vi "New Project.vi"(9 "DBSet":T1={"Server"="172.20.23.107", "DB"="HTPSDB", "PSW"="data'songyy", "User"="sa"}, 10 "UserID":string="L043460", 11 "厂区":string="清溪") -> ()   [LabVIEW 2011] (continued)
                                n506 = local read "Luxshare_P/N:"() -> (w621:string)
                                n507 = local read "Luxshare_P/N:"() -> (w624:string)
                                n508 = local read "Luxshare_P/N:"() -> (w627:string)
                                n509 = local read "厂区"() -> ()  [unwired: 1 out]
                                n510 = local read "厂区"() -> (w583:string)
                                n511 = call "query.net.vi"() -> ()  [unwired: 10 in, 2 out]
                                n512 = call "_wmg_PNtoPNwhereConnect.vi"("Input"=w621) -> ("Output"=w595:string)
                                n513 = call "_wmg_PNtoPNwhereConnect.vi"("Input"=w627) -> ("Output"=w600:string)
                                n514 = call "_wmg_PNtoPNwhereConnect.vi"("Input"=w624) -> ("Output"=w598:string)
                                n515 = property on="System_Mode" class="Ring (严格)"() -> ("RingText.Text"=w594:string)  [unwired: 2 in, 2 out]
                                n516 = call "_wmg_HardModetoHardModewhereConnect.vi"("Input"=w594, "Factory"=w583) -> ("Output"=w585:string)
                                n517 = Concatenate Strings(w600, w585) -> (w599:string)
                                n518 = call "sql-readinfo_vproject.vi"("DBSet"=w582, "操作模式"=T7."查询数据", "查询项目"="Prjinf", "限定条件"=w599) -> ("ResultString"=w614:string)  [unwired: 13 in, 10 out]
                                n519 = local write "Project Information"(w614) -> ()
                                n520 = Concatenate Strings(w595, w585) -> (w593:string)
                                n521 = call "sql-readinfo_vproject.vi"("DBSet"=w582, "操作模式"=T7."查询数据", "查询项目"="SwitchMatrix", "限定条件"=w593) -> ("ResultString"=w616:string)  [unwired: 13 in, 10 out]
                                n522 = Concatenate Strings(w598, w585) -> (w597:string)
                                n523 = call "sql-readinfo_vproject.vi"("DBSet"=w582, "操作模式"=T7."查询数据", "查询项目"="Spec", "限定条件"=w597) -> ("ResultString"=→"Spec_midVar":string)  [unwired: 13 in, 10 out]
                                n524 = local write "Switch Matrix"(w616) -> ()
                                n525 = local read "Luxshare_P/N:"() -> (w606:string)
                                n526 = local read "Luxshare_P/N:"() -> (w609:string)
                                n527 = local read "Luxshare_P/N:"() -> (w612:string)
                                n528 = local read "Luxshare_P/N:"() -> (w618:string)
                                n529 = call "_wmg_PNtoPNwhereConnect.vi"("Input"=w606) -> ("Output"=w586:string)
                                n530 = Concatenate Strings(w586, w585) -> (w584:string)
                                n531 = call "_wmg_PNtoPNwhereConnect.vi"("Input"=w609) -> ("Output"=w588:string)
                                n532 = Concatenate Strings(w588, w585) -> (w587:string)
                                n533 = call "_wmg_PNtoPNwhereConnect.vi"("Input"=w612) -> ("Output"=w590:string)
                                n534 = Concatenate Strings(w590, w585) -> (w589:string)
                                n535 = call "sql-readinfo_vproject.vi"("DBSet"=w582, "操作模式"=T7."查询数据", "查询项目"="Spec_Points", "限定条件"=w584) -> ("ResultString"=w602:string)  [unwired: 13 in, 10 out]
                                n536 = call "sql-readinfo_vproject.vi"("DBSet"=w582, "操作模式"=T7."查询数据", "查询项目"="Switch_File_Path", "限定条件"=w589) -> ("ResultString"=w604:string)  [unwired: 13 in, 10 out]
                                n537 = call "_wmg_PNtoPNwhereConnect.vi"("Input"=w618) -> ("Output"=w592:string)
                                n538 = Concatenate Strings(w592, w585) -> (w591:string)
                                n539 = call "sql-readinfo_vproject.vi"("DBSet"=w582, "操作模式"=T7."查询数据", "查询项目"="LabelC", "限定条件"=w591) -> ("ResultString"=w615:string)  [unwired: 13 in, 10 out]
                                n540 = call "sql-readinfo_vproject.vi"("DBSet"=w582, "操作模式"=T7."查询数据", "查询项目"="Spec_File_Path", "限定条件"=w587) -> ("ResultString"=w603:string)  [unwired: 13 in, 10 out]
                                n541 = Decimal String To Number(string=w602) -> (number=w601:i32)  [unwired: 2 in, 1 out]
                                n542 = local write "Spec Points"(w601) -> ()
                                n543 = local write "Spec File Path"(w603) -> ()
                                n544 = local write "Switch File Path"(w604) -> ()
                                n545 = local write "Label Content"(w615) -> ()
                              }
                              frame Enabled {
                              }
                            }
                          }
                          frame #3 {
                            n546 = local read "Luxshare_P/N:"() -> (w644:string)
                            n547 = property on="System_Mode" class="Ring (严格)"() -> ("RingText.Text"=w643:string)  [unwired: 2 in, 2 out]
                            n548 = local read "厂区"() -> (w642:string)
                            n549 = Search and Replace String(input string="select SwitchMatrix ,Prjinf,Spec,LabelC,Switch_File_Path,Spec_File_Path,Spec_Points from vproject where LuxsharePN='@PN@' and HardWare_Mode='@Mode@' and  Factory ='@Facotry@'", search string="@PN@" ("搜索字符串"), replace string=w644) -> (result string=w648:string)  [unwired: 5 in, 3 out]
                            n550 = Search and Replace String(input string=w648, search string="@Mode@" ("搜索字符串"), replace string=w643) -> (result string=w646:string)  [unwired: 5 in, 3 out]
                            n551 = Search and Replace String(input string=w646, search string="@Facotry@" ("搜索字符串"), replace string=w642) -> (result string=w641:string)  [unwired: 5 in, 3 out]
                            n552 = call "query.net.vi"("Sql"=w641, "DBSet"=w640) -> ("result"=w639:string[][])  [unwired: 8 in, 1 out]
                            n553 = Index Array(array=w639, index (row)=0 ("索引 (行)")) -> (element=w637:string[])  [unwired: 1 in]
                            n554 = Index Array(array=w637) -> (element #1=w636:string, element #2=w635:string, element #3=w634:string, element #4=w633:string, element #5=w632:string, element #6=w631:string, element #7=w630:string)  [unwired: 7 in]
                            n555 = Decimal String To Number(string=w630) -> (number=w629:i32)  [unwired: 2 in, 1 out]
                            n556 = local write "Switch Matrix"(w636) -> ()
                            n557 = local write "Project Information"(w635) -> ()
                            n558 = local write "Spec_midVar"(w634) -> ()
                            n559 = local write "Label Content"(w633) -> ()
                            n560 = local write "Switch File Path"(w632) -> ()
                            n561 = local write "Spec File Path"(w631) -> ()
                            n562 = local write "Spec Points"(w629) -> ()
                          }
                          frame #4 {
                            n563 = control-ref of="Cable AWG:"() -> (w651:refnum<vi>)
                            n564 = local read "Spec_midVar"() -> (w654:string)
                            n565 = Search and Replace String(replace all?=TRUE ("替换全部？(F)"), input string=w654, search string="#" ("搜索字符串"), replace string="\t") -> (result string=w658:string)  [unwired: 4 in, 3 out]
                            n566 = control-ref of="Customer"() -> (w652:refnum<vi>)
                            n567 = local read "Customer"() -> (w665:string)
                            n568 = local read "AWG"() -> (w664:string)
                            n569 = Spreadsheet String To Array(format string="%s" ("格式字符串"), spreadsheet string=w658, array type (2D Dbl)=string[][] []) -> (array=w653:string[][])  [unwired: 1 in]
                            n570 = call "_wmg_downlistValue.vi"("Customer"=w664, "CustomerRef"=w651) -> ()  [unwired: 1 in]
                            n571 = call "_wmg_downlistValue.vi"("Customer"=w665, "CustomerRef"=w652) -> ()  [unwired: 1 in]
                            n572 = Array To Spreadsheet String(delimiter (Tab)="#" ("分隔符(Tab)"), array=w653, 3:"%s" ("格式字符串")) -> (spreadsheet string=w663:string)
                            n573 = local write "Spec Associate"(w653) -> ()
                            n574 = local write "Spec String"(w663) -> ()
                          }
                        }
                      }
                    }
                  }
                  frame #1 {
                    # "列数\n0. S-para Pair Name\n1. NEXT Pair Name\n2. FEXT Pair Name\n3. Diff TestItems\n4. Single TestItems\n5. TDR TestItems\n6. Spec Associate\n7. VNA Cal File Path\n8. Report Config\n9. ILD Spec\n10. TDR Setting"
                    # "解析Prjinf"
                    n575 = local read "Project Information"() -> (w700:string)
                    n576 = Spreadsheet String To Array(delimiter (Tab)="#" ("分隔符(Tab)"), format string="%s" ("格式字符串"), spreadsheet string=w700, array type (2D Dbl)=string[][] []) -> (array=w697:string[][])
                    n577 = Index Array(array=w697, index (col) #1=0 ("索引"), index (col) #2=1 ("索引 (列)"), index (col) #3=2 ("索引 (列)"), index (col) #4=3 ("索引 (列)"), index (col) #5=4 ("索引 (列)"), index (col) #6=5 ("索引"), index (col) #7=6 ("索引 (列)"), index (col) #8=7 ("索引 (列)"), index (col) #9=8 ("索引 (列)"), index (col) #10=9 ("索引 (列)"), index (col) #11=10 ("索引"), index (col) #12=11 ("索引 (列)"), index (col) #13=12 ("索引 (列)"), index (col) #14=13 ("索引 (列)"), index (col) #15=14 ("索引 (列)")) -> (element #1=w696:string[], element #2=w695:string[], element #3=w694:string[], element #4=w693:string[], element #5=w692:string[], element #6=w691:string[], element #7=w690:string[], element #8=w689:string[], element #9=w688:string[], element #10=w687:string[], element #11=w686:string[], element #12=w673:string[], element #13=w670:string[], element #14=w668:string[], element #15=w666:string[])  [unwired: 15 in]
                    n578 = stacked-sequence {
                      tunnel: w696 -> [_ w714 _ _ _ _ _ _ _]
                      tunnel: w695 -> [_ w713 _ _ _ _ _ _ _]
                      tunnel: w694 -> [_ w712 _ _ _ _ _ _ _]
                      tunnel: w693 -> [_ w711 _ _ _ _ _ _ _]
                      tunnel: w692 -> [_ w710 _ _ _ _ _ _ _]
                      tunnel: w691 -> [_ w709 _ _ _ _ _ _ _]
                      tunnel: w690 -> [_ _ w760 _ _ _ _ _ _]
                      tunnel: w689 -> [_ _ w759 _ _ _ _ _ _]
                      tunnel: w688 -> [_ _ _ w788 _ _ _ _ _]
                      tunnel: w687 -> [_ _ _ _ _ _ _ _ _]
                      tunnel: w686 -> [_ _ _ _ _ w808 _ _ _]
                      tunnel: w673 -> [_ _ _ _ _ _ w838 _ _]
                      tunnel: w670 -> [_ _ _ w780 _ _ _ _ _]
                      tunnel: w668 -> [_ _ _ _ _ _ _ w882 _]
                      tunnel: w666 -> [_ _ _ _ _ _ _ _ w889]
                      frame #0 {
                        n579 = local read "Single init"() -> (→"Single init 2":i32[])
                        n580 = local read "NEXT init"() -> (→"NEXT init 2":i32[])
                        n581 = local read "FEXT init"() -> (→"FEXT init 2":i32[])
                        n582 = local read "S-p init"() -> (→"S-p init 2":i32[])
                        n583 = local read "Diff init"() -> (→"Diff init 2":i32[])
                        n584 = local read "TDR init"() -> (→"TDR init 2":i32[])
                      }
                      frame #1 {
                        n585 = stacked-sequence {
                          tunnel: [_ w736 _ _] -> _
                          tunnel: w714 -> [_ w736 _ _]
                          tunnel: w713 -> [_ w729 _ _]
                          tunnel: w712 -> [_ _ w742 _]
                          tunnel: w711 -> [_ _ w737 _]
                          tunnel: w710 -> [_ _ _ w750]
                          tunnel: w709 -> [_ _ _ w747]
                          frame #0 {
                            n586 = local read "FEXT init"() -> (w722:string[])
                            n587 = local read "FEXT init"() -> (w721:i32[])
                            n588 = local read "NEXT init"() -> (w725:string[])
                            n589 = local read "NEXT init"() -> (w723:i32[])
                            n590 = local read "S-p init"() -> (w724:i32[])
                            n591 = local read "S-p init"() -> (w726:string[])
                            n592 = property on="S-para Pair Name" class="LstBox (严格)"("Item Names"=w726, "Item Symbols"=w724) -> ()  [unwired: 2 in, 2 out]
                            n593 = property on="NEXT Pair Name" class="LstBox (严格)"("Item Names"=w725, "Item Symbols"=w723) -> ()  [unwired: 2 in, 2 out]
                            n594 = property on="FEXT Pair Name" class="LstBox (严格)"("Item Names"=w722, "Item Symbols"=w721) -> ()  [unwired: 2 in, 2 out]
                            n595 = local read "Single init"() -> (w718:string[])
                            n596 = local read "Single init"() -> (w717:i32[])
                            n597 = local read "TDR init"() -> (w716:string[])
                            n598 = local read "TDR init"() -> (w715:i32[])
                            n599 = local read "Diff init"() -> (w720:string[])
                            n600 = local read "Diff init"() -> (w719:i32[])
                            n601 = property on="Diff Test Items" class="LstBox (严格)"("Item Names"=w720, "Item Symbols"=w719) -> ()  [unwired: 2 in, 2 out]
                            n602 = property on="Single Test Items" class="LstBox (严格)"("Item Names"=w718, "Item Symbols"=w717) -> ()  [unwired: 2 in, 2 out]
                            n603 = property on="TDR Test Items" class="LstBox (严格)"("Item Names"=w716, "Item Symbols"=w715) -> ()  [unwired: 2 in, 2 out]
                          }
                          frame #1 {
                            n604 = local read "S-p init"() -> (w734:i32[])
                            n605 = local read "NEXT init"() -> (w727:string[])
                            n606 = local read "NEXT init"() -> (w730:i32[])
                            n607 = local read "S-p init"() -> (w728:string[])
                            n608 = call "_wmg_readItems.vi"("input_p"=w734, "input"=w728, "input_sp"=w736) -> ("output_p"=w733:i32[], "output_sp"=w735:string[])
                            n609 = call "_wmg_readItems2.vi"("input_p"=w730, "input"=w727, "input_sp"=w729) -> ("output_p"=w731:i32[], "output_sp"=w732:string[])
                            n610 = property on="S-para Pair Name" class="LstBox (严格)"("Item Names"=w735, "Item Symbols"=w733) -> ()  [unwired: 2 in, 2 out]
                            n611 = property on="NEXT Pair Name" class="LstBox (严格)"("Item Names"=w732, "Item Symbols"=w731) -> ()  [unwired: 2 in, 2 out]
                          }
                          frame #2 {
                            n612 = local read "FEXT init"() -> (w745:string[])
                            n613 = local read "FEXT init"() -> (w746:i32[])
                            n614 = local read "Diff init"() -> (w741:string[])
                            n615 = local read "Diff init"() -> (w740:i32[])
                            n616 = call "_wmg_readItems2.vi"("input_p"=w740, "input"=w741, "input_sp"=w737) -> ("output_p"=w739:i32[], "output_sp"=w738:string[])
                            n617 = call "_wmg_readItems.vi"("input_p"=w746, "input"=w745, "input_sp"=w742) -> ("output_p"=w743:i32[], "output_sp"=w744:string[])
                            n618 = property on="FEXT Pair Name" class="LstBox (严格)"("Item Names"=w744, "Item Symbols"=w743) -> ()  [unwired: 2 in, 2 out]
                            n619 = property on="Diff Test Items" class="LstBox (严格)"("Item Names"=w738, "Item Symbols"=w739) -> ()  [unwired: 2 in, 2 out]
                          }
                          frame #3 {
                            n620 = local read "TDR init"() -> (w749:string[])
                            n621 = local read "TDR init"() -> (w748:i32[])
                            n622 = local read "Single init"() -> (w751:string[])
                            n623 = local read "Single init"() -> (w752:i32[])
                            n624 = call "_wmg_readItems.vi"("input_p"=w752, "input"=w751, "input_sp"=w750) -> ("output_p"=w754:i32[], "output_sp"=w753:string[])
                            n625 = call "_wmg_readItems2.vi"("input_p"=w748, "input"=w749, "input_sp"=w747) -> ("output_p"=w756:i32[], "output_sp"=w755:string[])
                            n626 = property on="TDR Test Items" class="LstBox (严格)"("Item Names"=w755, "Item Symbols"=w756) -> ()  [unwired: 2 in, 2 out]
                            n627 = property on="Single Test Items" class="LstBox (严格)"("Item Names"=w753, "Item Symbols"=w754) -> ()  [unwired: 2 in, 2 out]
                          }
                        }
                      }
                      frame #2 {
                        n628 = disable-structure shown="禁用" {
                          disable-tunnel: w760 -> [w761 _]
                          frame Disabled {
                            n629 = property on="Diff Test Items" class="LstBox (严格)"() -> ("Item Symbols"=w765:i32[], "Item Names"=w763:string[])  [unwired: 2 in, 2 out]
                            n630 = for {
                              tunnel: w765 -> [w771] mode=indexing
                              shift-right: [w766] -> w762
                              shift-left: string[] [] -> [w767]
                              tunnel: w763 -> [w768] mode=indexing
                              n631 = Not Equal?(x=w771, y=37) -> (x != y?=w769:bool)
                              n632 = case shown="假" w769 {
                                tunnel: w768 -> [_ w775]
                                tunnel: w767 -> [w772 w774]
                                tunnel: [w772 w773] -> w766
                                frame False {
                                }
                                frame True {
                                n633 = Insert Into Array(array=w774, new element=w775) -> (w773:string[])  [unwired: 1 in]
                                }
                              }
                            }
                            n634 = Build Array(w762, w761) -> ()  [unwired: 1 out]
                          }
                          frame Enabled {
                          }
                        }
                        n635 = Index Array(array=w759, index=0 ("索引")) -> (element=w758:string)
                        n636 = local write "VNA Cal File Path:"(w758) -> ()
                      }
                      frame #3 {
                        n637 = Index Array(array=w780, index=0 ("索引")) -> (element=w778:string)
                        n638 = Index Array(array=w788, index #1=0 ("索引"), index #3=2 ("索引")) -> (element #1=w785:string, element #2=w784:string, element #3=w782:string)  [unwired: 1 in]
                        n639 = Equal?(x=w778, y="TRUE") -> (x = y?=w776:bool)
                        n640 = String To Path(string=w785) -> (path=w786:path)
                        n641 = call "_wmg_ReportConfigDivided@.vi"("Input"=w784) -> ("Output"=w783:string[][])
                        n642 = call "_wmg_ReportConfigDivided@.vi"("Input"=w782) -> ("Output"=w781:string[][])
                        n643 = local write "Postion for Raw data"(w783) -> ()
                        n644 = local write "Report Templete Path:"(w786) -> ()
                        n645 = local write "Postion for \"PN&Tester&Date\" etc Fields"(w781) -> ()
                        n646 = local write "Cancel Dem2X?"(w776) -> ()
                      }
                      frame #4 {
                      }
                      frame #5 {
                        # "TDR Setting\n0. Start TimeNs\n1. Stop TimeNs\n2. Data Points\n3. Filter Risetime(ps)\n4. Compensation(ohm)\n5. Impedance Filter\n6. Impedance Spec:\n7. Delay Spec:\n8. skew Spec:\n9. IL 2X Data:"
                        n647 = Index Array(array=w808, index #1=0 ("索引"), index #2=1 ("索引"), index #3=2 ("索引"), index #4=3 ("索引"), index #5=4 ("索引"), index #6=5 ("索引"), index #7=6 ("索引"), index #8=9 ("索引"), index #9=8 ("索引")) -> (element #1=w800:string, element #2=w799:string, element #3=w798:string, element #4=w797:string, element #5=w796:string, element #6=w795:string, element #7=w794:string, element #8=w792:string, element #9=w790:string)
                        n648 = stacked-sequence {
                          tunnel: w800 -> [w835]
                          tunnel: w799 -> [w832]
                          tunnel: w798 -> [w830]
                          tunnel: w797 -> [w829]
                          tunnel: w796 -> [w826]
                          tunnel: w795 -> [w825]
                          tunnel: w794 -> [w822]
                          tunnel: w792 -> [w817]
                          tunnel: w790 -> [w811]
                          frame #0 {
                            n649 = call "_wmg_ImpSpecDivided@.vi"("Input"=w822) -> ("Output"=w821:string[][])
                            n650 = Spreadsheet String To Array(format string="%s" ("格式字符串"), spreadsheet string=w817, array type (2D Dbl)=dbl[] []) -> (array=w812:dbl[])  [unwired: 1 in]
                            n651 = Fract/Exp String To Number(string=w811) -> (number=w810:dbl)  [unwired: 3 in, 1 out]
                            n652 = local write "Skew max(ps)"(w810) -> ()
                            n653 = Insert Into Array(array=w821, index (col)=0 ("禁用的索引 (列)"), new element=string[] ["Mating Area", "Cable Area", "Cable End"]) -> (w819:string[][])  [unwired: 1 in]
                            n654 = local write "2X Thru  IL Data"(w812) -> ()
                            n655 = Decimal String To Number(string=w825) -> (number=w809:i32)  [unwired: 2 in, 1 out]
                            n656 = local write "Impedance Spec:"(w819) -> ()
                            n657 = Number To Boolean Array(number=w809) -> (Boolean array=w824:bool[])
                            n658 = Array To Spreadsheet String(array=w812, 3:"%s" ("格式字符串")) -> (spreadsheet string=w814:string)  [unwired: 1 in]
                            n659 = Fract/Exp String To Number(string=w826) -> (number=w827:dbl)  [unwired: 3 in, 1 out]
                            n660 = Index Array(array=w824) -> (element=w823:bool)  [unwired: 1 in]
                            n661 = Fract/Exp String To Number(string=w832) -> (number=w833:dbl)  [unwired: 3 in, 1 out]
                            n662 = Decimal String To Number(string=w830) -> (number=w831:i32)  [unwired: 2 in, 1 out]
                            n663 = Fract/Exp String To Number(string=w829) -> (number=w828:dbl)  [unwired: 3 in, 1 out]
                            n664 = local write "2X Thru String"(w814) -> ()
                            n665 = local write "Compensation(ohm)"(w827) -> ()
                            n666 = Fract/Exp String To Number(string=w835) -> (number=w834:dbl)  [unwired: 3 in, 1 out]
                            n667 = local write "Filter Risetime(ps)"(w828) -> ()
                            n668 = local write "Impedance Filter"(w823) -> ()
                            n669 = local write "Start TimeNs"(w834) -> ()
                            n670 = local write "StopTimeNs"(w833) -> ()
                            n671 = local write "Data Points"(w831) -> ()
                          }
                        }
                      }
                      frame #6 {
                        # "TDR Setting\n0. Start TimeNs\n1. Stop TimeNs\n2. Data Points\n3. Filter Risetime(ps)\n4. Compensation(ohm)\n5. Impedance Filter\n6. Impedance Spec:\n7. Delay Spec:\n8. skew Spec:\n9. IL 2X Data:"
                        n672 = Index Array(array=w838, index #1=0 ("索引"), index #2=1 ("索引"), index #3=2 ("索引"), index #4=3 ("索引"), index #5=4 ("索引"), index #6=5 ("索引"), index #7=6 ("索引"), index #8=9 ("索引"), index #9=8 ("索引")) -> (element #1=w847:string, element #2=w846:string, element #3=w845:string, element #4=w844:string, element #5=w843:string, element #6=w842:string, element #7=w841:string, element #8=w839:string, element #9=w836:string)
                        n673 = stacked-sequence {
                          tunnel: w847 -> [w878]
                          tunnel: w846 -> [w877]
                          tunnel: w845 -> [w876]
                          tunnel: w844 -> [w875]
                          tunnel: w843 -> [w874]
                          tunnel: w842 -> [w873]
                          tunnel: w841 -> [w871]
                          tunnel: w839 -> [w868]
                          tunnel: w836 -> [w858]
                          frame #0 {
                            (unwired) string[] ["Mating Area", "Cable Area"]
                            n674 = call "_wmg_ImpSpecDivided@.vi"("Input"=w871) -> ("Output"=w870:string[][])
                            n675 = Spreadsheet String To Array(format string="%s" ("格式字符串"), spreadsheet string=w868, array type (2D Dbl)=dbl[] []) -> ()  [unwired: 1 in, 1 out]
                            n676 = Fract/Exp String To Number(string=w858) -> (number=w857:dbl)  [unwired: 3 in, 1 out]
                            n677 = local write "Skew max(ps) 2"(w857) -> ()
                            n678 = Insert Into Array(array=w870, index (col)=0 ("禁用的索引 (列)"), new element=string[] ["Mating Area", "Cable Area", "Cable End"]) -> (w865:string[][])  [unwired: 1 in]
                            n679 = Decimal String To Number(string=w873) -> (number=w856:i32)  [unwired: 2 in, 1 out]
                            n680 = local write "Impedance Spec: 2"(w865) -> ()
                            n681 = Number To Boolean Array(number=w856) -> (Boolean array=w872:bool[])
                            n682 = Fract/Exp String To Number(string=w874) -> (number=w863:dbl)  [unwired: 3 in, 1 out]
                            n683 = Index Array(array=w872) -> (element=w864:bool)  [unwired: 1 in]
                            n684 = Fract/Exp String To Number(string=w877) -> (number=w860:dbl)  [unwired: 3 in, 1 out]
                            n685 = Decimal String To Number(string=w876) -> (number=w861:i32)  [unwired: 2 in, 1 out]
                            n686 = Fract/Exp String To Number(string=w875) -> (number=w862:dbl)  [unwired: 3 in, 1 out]
                            n687 = local write "Compensation(ohm) 2"(w863) -> ()
                            n688 = Fract/Exp String To Number(string=w878) -> (number=w859:dbl)  [unwired: 3 in, 1 out]
                            n689 = local write "Filter Risetime(ps) 2"(w862) -> ()
                            n690 = local write "Impedance Filter 2"(w864) -> ()
                            n691 = local write "Data Points 2"(w861) -> ()
                            n692 = local write "StopTimeNs 2"(w860) -> ()
                            n693 = local write "Start TimeNs 2"(w859) -> ()
                          }
                        }
                      }
                      frame #7 {
                        n694 = Index Array(array=w882, index=0 ("索引")) -> (element=w880:string)
                        n695 = Decimal String To Number(string=w880) -> (number=w879:i32)  [unwired: 2 in, 1 out]
                        n696 = local write "平滑点数"(w879) -> ()
                      }
                      frame #8 {
                        n697 = Index Array(array=w889, index=0 ("索引")) -> (element=w887:string)
                        n698 = call "_wmg_ImpSpecDivided@.vi"("Input"=w887) -> ("Output"=w886:string[][])
                        n699 = Insert Into Array(array=w886, index (col)=0 ("禁用的索引 (列)"), new element=string[] ["Mating Area", "Cable Area", "Cable End"]) -> (w883:string[][])  [unwired: 1 in]
                        n700 = local write "Common Impedance Spec"(w883) -> ()
                      }
                    }
                    n701 = disable-structure shown="禁用" {
                      frame Disabled {
                        n702 = local read "2X Thru  IL Data"() -> ()  [unwired: 1 in]
                        n703 = Array To Spreadsheet String(3:"%s" ("格式字符串")) -> (spreadsheet string=w701:string)  [unwired: 2 in]
                        n704 = local write "2X Thru String"(w701) -> ()
                      }
                      frame Enabled {
                      }
                    }
                  }
                  frame #2 {
                    w898 = T4 {"Row"=0, "Column"=0} ("编辑位置")
                    w899 = u32 4 ("列数")
                    n705 = property on="Single Test Items" class="LstBox (严格)"() -> ("Item Names"=w906:string[], "Item Symbols"=w905:i32[])  [unwired: 2 in, 2 out]
                    n706 = property on="TDR Test Items" class="LstBox (严格)"() -> ("Item Names"=w904:string[], "Item Symbols"=w903:i32[])  [unwired: 2 in, 2 out]
                    n707 = property on="Diff Test Items" class="LstBox (严格)"() -> ("Item Names"=w908:string[], "Item Symbols"=w907:i32[])  [unwired: 2 in, 2 out]
                    n708 = call "_wmg_SelectItems2.vi"("Item Syms"=w903, "Item name"=w904) -> ("Selected tem"=w902:string[])  [unwired: 7 in, 2 out]
                    n709 = call "_wmg_SelectItems2.vi"("Item Syms"=w907, "Item name"=w908) -> ("Selected tem"=w901:string[])  [unwired: 7 in, 2 out]
                    n710 = call "_wmg_SelectItems2.vi"("Item Syms"=w905, "Item name"=w906) -> ("Selected tem"=w900:string[])  [unwired: 7 in, 2 out]
                    n711 = property on="Postion for Raw data" class="Tbl (严格)"() -> ("Value"=w897:string[][])  [unwired: 2 in, 2 out]
                    n712 = Insert Into Array(array=w902, new element #1=w901, new element #2=w900) -> (w896:string[])  [unwired: 1 in]
                    n713 = local read "2X Thru  IL Data"() -> (w892:dbl[])
                    n714 = Replace Array Subset(array=w897, new element=w896, index (col)=0 ("禁用的索引 (列)")) -> (w895:string[][])  [unwired: 1 in]
                    n715 = property on="Postion for Raw data" class="Tbl (严格)"("Value"=w895) -> ()  [unwired: 2 in, 2 out]
                    n716 = Array Size(array=w892) -> (size(s)=w891:i32)
                    n717 = for {
                      N: w891 -> [_]
                      tunnel: [w909] -> w890 mode=indexing
                      i -> [w909]
                    }
                    n718 = Bundle(w890, "2X Thru  IL Data"=w892) -> (w893:cluster{i32[], "2X Thru  IL Data":dbl[]})  [unwired: 1 in]
                    n719 = local write "Insertion Loss"(w893) -> ()
                    n720 = property on="Postion for Raw data" class="Tbl (严格)"("Number of Columns"=w899, "EditPos"=w898) -> ()  [unwired: 2 in, 2 out]
                    n721 = property on="Postion for \"PN&Tester&Date\" etc Fields" class="Tbl (严格)"("Number of Columns"=w899, "EditPos"=w898) -> ()  [unwired: 2 in, 2 out]
                  }
                  frame #3 {
                    n722 = local read "Local"() -> (w910:bool)
                    n723 = case shown="真" w910 {
                      frame False {
                        n724 = local read "result_query"() -> (w914:string)
                        n725 = call <vilib>:"Trim Whitespace.vi"("string"=w914) -> ("trimmed string"=w913:string)  [unwired: 1 in]
                        n726 = String Length(string=w913) -> (length=w912:i32)
                        n727 = Equal To 0?(x=w912) -> (x = 0?=w911:bool)
                        n728 = case shown="假" w911 {
                          frame False {
                            n729 = property on="Update" class="Bool (严格)"("DisabledEnum"=T5."Enabled" ("禁用")) -> ()  [unwired: 2 in, 2 out]
                            n730 = property on="Delete" class="Bool (严格)"("DisabledEnum"=T5."Enabled" ("禁用")) -> ()  [unwired: 2 in, 2 out]
                          }
                          frame True {
                            n731 = local write "Luxshare_P/N:"("") -> ()
                            n732 = One Button Dialog(message="数据库中无此记录" ("消息")) -> ()  [unwired: 1 in, 1 out]
                          }
                        }
                      }
                      frame True {
                        n733 = local read "fileexist"() -> (w920:bool)
                        n734 = Not(x=w920) -> (.not. x?=w919:bool)
                        n735 = case shown="假" w919 {
                          frame False {
                            # "文件不存在"
                            n736 = local read "Impedance Spec:"() -> (w924:string[][])
                            n737 = local write "Luxshare_P/N:"("") -> ()
                            n738 = Replace Array Subset(array=w924, new element=string[] ["", "", ""] ("新元素/子数组"), index (col)=0 ("禁用的索引 (列)")) -> (w923:string[][])  [unwired: 1 in]
                            n739 = local write "Impedance Spec:"(w923) -> ()
                            n740 = property on="Update" class="Bool (严格)"("DisabledEnum"=T5."Disabled and Grayed Out" ("禁用")) -> ()  [unwired: 2 in, 2 out]
                            n741 = property on="Delete" class="Bool (严格)"("DisabledEnum"=T5."Disabled and Grayed Out" ("禁用")) -> ()  [unwired: 2 in, 2 out]
                          }
                          frame True {
                            n742 = property on="Update" class="Bool (严格)"("DisabledEnum"=T5."Enabled" ("禁用")) -> ()  [unwired: 2 in, 2 out]
                            n743 = property on="Delete" class="Bool (严格)"("DisabledEnum"=T5."Enabled" ("禁用")) -> ()  [unwired: 2 in, 2 out]
                          }
                        }
                      }
                    }
                  }
                }
              }
              frame 100 {
                # "updata"
                n744 = stacked-sequence {
                  tunnel: w930 -> [w931 w950 _]
                  frame #0 {
                    n745 = local read "Local"() -> (w932:bool)
                    n746 = case shown="真" w932 {
                      tunnel: w931 -> [w943 _]
                      frame False {
                        n747 = local read "Luxshare_P/N:"() -> (w935:string)
                        n748 = Search and Replace String(input string="delete from vproject where LuxsharePN='@PN@' and HardWare_Mode='@Mode@' and  Factory ='@Facotry@'", search string="@PN@" ("搜索字符串"), replace string=w935) -> (result string=w941:string)  [unwired: 5 in, 3 out]
                        n749 = property on="System_Mode" class="Ring (严格)"() -> ("RingText.Text"=w934:string)  [unwired: 2 in, 2 out]
                        n750 = Search and Replace String(input string=w941, search string="@Mode@" ("搜索字符串"), replace string=w934) -> (result string=w939:string)  [unwired: 5 in, 3 out]
                        n751 = local read "厂区"() -> (w933:string)
                        n752 = Search and Replace String(input string=w939, search string="@Facotry@" ("搜索字符串"), replace string=w933) -> (result string=w936:string)  [unwired: 5 in, 3 out]
                        n753 = call "query.net.vi"("Sql"=w936, "DBSet"=w943) -> ()  [unwired: 8 in, 2 out]
                      }
                      frame True {
                        n754 = local read "Luxshare_P/N:"() -> (w945:string)
                        n755 = call <vilib>:"Application Directory.vi"() -> ("Application Directory"=w949:path)
                        n756 = Concatenate Strings("Database\\" ("字符串"), w945, ".hpj" ("字符串")) -> (w948:string)
                        n757 = Build Path(base path=w949, name or relative path=w948) -> (appended path=w944:path)
                        n758 = Delete(path (use dialog)=w944) -> ()  [unwired: 4 in, 3 out]
                      }
                    }
                  }
                  frame #1 {
                    n759 = stacked-sequence {
                      tunnel: w950 -> [_ _ _ _ w1134 _]
                      frame #0 {
                        w980 = "@"
                        w981 = "\r\n"
                        w990 = "%s" ("格式字符串")
                        n760 = local read "Impedance Filter"() -> (w967:bool)
                        n761 = local read "Impedance Spec:"() -> (w992:string[][])
                        n762 = local read "2X Thru String"() -> (w977:string)
                        n763 = property on="Skew max(ps)" class="DigNum (严格)"() -> ("NumText.Text"=w969:string)  [unwired: 2 in, 2 out]
                        n764 = property on="Delay(ns)" class="DigNum (严格)"() -> ("NumText.Text"=w976:string)  [unwired: 2 in, 2 out]
                        n765 = property on="Start TimeNs" class="DigNum (严格)"() -> ("NumText.Text"=w975:string)  [unwired: 2 in, 2 out]
                        n766 = property on="StopTimeNs" class="DigNum (严格)"() -> ("NumText.Text"=w974:string)  [unwired: 2 in, 2 out]
                        n767 = property on="Data Points" class="DigNum (严格)"() -> ("NumText.Text"=w973:string)  [unwired: 2 in, 2 out]
                        n768 = property on="Filter Risetime(ps)" class="DigNum (严格)"() -> ("NumText.Text"=w972:string)  [unwired: 2 in, 2 out]
                        n769 = property on="Compensation(ohm)" class="DigNum (严格)"() -> ("NumText.Text"=w971:string)  [unwired: 2 in, 2 out]
                        n770 = Boolean To (0,1)(Boolean=w967) -> (0, 1=w994:i16)
                        n771 = Number To Decimal String(number=w994) -> (decimal integer string=w993:string)  [unwired: 1 in]
                        n772 = call "impedance spec.vi"("Impedance Spec:"=w992) -> ("Impedance spec string"=w991:string)  [unwired: 10 in]
                        n773 = call <vilib>:"Trim Whitespace.vi"("string"=w977) -> ("trimmed string"=w966:string)  [unwired: 1 in]
                        n774 = Build Array(w975, w974, w973, w972, w971, w993, w991, w976, w969, w966) -> (w970:string[])
                        n775 = local read "2X Thru String"() -> (w964:string)
                        n776 = local read "Report Templete Path:"() -> (w978:path)
                        n777 = property on="Postion for Raw data" class="Tbl (严格)"() -> ("Value"=w989:string[][])  [unwired: 2 in, 2 out]
                        n778 = local write "TDR Setting"(w970) -> ()
                        n779 = property on="Postion for \"PN&Tester&Date\" etc Fields" class="Tbl (严格)"() -> ("Value"=w988:string[][])  [unwired: 2 in, 2 out]
                        n780 = local read "Impedance Filter 2"() -> (w951:bool)
                        n781 = Array To Spreadsheet String(array=w989, 3:w990) -> (spreadsheet string=w986:string)  [unwired: 1 in]
                        n782 = Array To Spreadsheet String(array=w988, 3:w990) -> (spreadsheet string=w984:string)  [unwired: 1 in]
                        n783 = local read "Impedance Spec: 2"() -> (w957:string[][])
                        n784 = Path To String(path=w978) -> (string=w979:string)
                        n785 = property on="Delay(ns)" class="DigNum (严格)"() -> ("NumText.Text"=w955:string)  [unwired: 2 in, 2 out]
                        n786 = property on="Skew max(ps) 2" class="DigNum (严格)"() -> ("NumText.Text"=w954:string)  [unwired: 2 in, 2 out]
                        n787 = property on="Start TimeNs 2" class="DigNum (严格)"() -> ("NumText.Text"=w963:string)  [unwired: 2 in, 2 out]
                        n788 = property on="StopTimeNs 2" class="DigNum (严格)"() -> ("NumText.Text"=w962:string)  [unwired: 2 in, 2 out]
                        n789 = property on="Data Points 2" class="DigNum (严格)"() -> ("NumText.Text"=w961:string)  [unwired: 2 in, 2 out]
                        n790 = property on="Filter Risetime(ps) 2" class="DigNum (严格)"() -> ("NumText.Text"=w960:string)  [unwired: 2 in, 2 out]
                        n791 = property on="Compensation(ohm) 2" class="DigNum (严格)"() -> ("NumText.Text"=w959:string)  [unwired: 2 in, 2 out]
                        n792 = Search and Replace String(replace all?=TRUE ("替换全部？(F)"), input string=w986, search string=w981, replace string=w980) -> (result string=w983:string)  [unwired: 4 in, 3 out]
                        n793 = Search and Replace String(replace all?=TRUE ("替换全部？(F)"), input string=w984, search string=w981, replace string=w980) -> (result string=w982:string)  [unwired: 4 in, 3 out]
                        n794 = Boolean To (0,1)(Boolean=w951) -> (0, 1=w965:i16)
                        n795 = Build Array(w979, w983, w982) -> (w968:string[])
                        n796 = Number To Decimal String(number=w965) -> (decimal integer string=w958:string)  [unwired: 1 in]
                        n797 = call "impedance spec.vi"("Impedance Spec:"=w957) -> ("Impedance spec string"=w956:string)  [unwired: 10 in]
                        n798 = call <vilib>:"Trim Whitespace.vi"("string"=w964) -> ("trimmed string"=w953:string)  [unwired: 1 in]
                        n799 = local write "Report Config"(w968) -> ()
                        n800 = Build Array(w963, w962, w961, w960, w959, w958, w956, w955, w954, w953) -> (w952:string[])
                        n801 = local write "TDR Setting2"(w952) -> ()
                      }
                      frame #1 {
                        n802 = local read "Common Impedance Spec"() -> (w998:string[][])
                        n803 = property on="S-para Pair Name" class="LstBox (严格)"() -> ("Item Names"=w1033:string[], "Item Symbols"=w1032:i32[])  [unwired: 2 in, 2 out]
                        n804 = property on="NEXT Pair Name" class="LstBox (严格)"() -> ("Item Names"=w1031:string[], "Item Symbols"=w1030:i32[])  [unwired: 2 in, 2 out]
                        n805 = property on="FEXT Pair Name" class="LstBox (严格)"() -> ("Item Names"=w1029:string[], "Item Symbols"=w1028:i32[])  [unwired: 2 in, 2 out]
                        n806 = property on="Single Test Items" class="LstBox (严格)"() -> ("Item Names"=w1035:string[], "Item Symbols"=w1034:i32[])  [unwired: 2 in, 2 out]
                        n807 = property on="Diff Test Items" class="LstBox (严格)"() -> ("Item Names"=w1037:string[], "Item Symbols"=w1036:i32[])  [unwired: 2 in, 2 out]
                        n808 = property on="TDR Test Items" class="LstBox (严格)"() -> ("Item Names"=w1015:string[], "Item Symbols"=w1014:i32[])  [unwired: 2 in, 2 out]
                        n809 = call "impedance spec.vi"("Impedance Spec:"=w998) -> ("Impedance spec string"=w997:string)  [unwired: 10 in]
                        n810 = call "Selected items.vi"("Item Syms"=w1032, "Item name"=w1033) -> ("Selected tem"=w1027:string[])  [unwired: 7 in, 2 out]
                        n811 = call "Selected items.vi"("Item Syms"=w1030, "Item name"=w1031) -> ("Selected tem"=w1026:string[])  [unwired: 7 in, 2 out]
                        n812 = call "Selected items.vi"("Item Syms"=w1028, "Item name"=w1029) -> ("Selected tem"=w1025:string[])  [unwired: 7 in, 2 out]
                        n813 = call "Selected items.vi"("Item Syms"=w1036, "Item name"=w1037) -> ("Selected tem"=w1024:string[])  [unwired: 7 in, 2 out]
                        n814 = call "Selected items.vi"("Item Syms"=w1034, "Item name"=w1035) -> ("Selected tem"=w1023:string[])  [unwired: 7 in, 2 out]
                        n815 = call "Selected items.vi"("Item Syms"=w1014, "Item name"=w1015) -> ("Selected tem"=w1013:string[])  [unwired: 7 in, 2 out]
                        n816 = Build Array(w997) -> (w996:string[])
                        n817 = local read "VNA Cal File Path:"() -> (w1010:string)
                        n818 = local read "ILD Spec"() -> (w1009:u16)
                        n819 = local read "Report Config"() -> (w1011:string[])
                        n820 = local read "TDR Setting2"() -> (w1007:string[])
                        n821 = local read "Cancel Dem2X?"() -> (w1006:bool)
                        n822 = local read "TDR Setting"() -> (w1012:string[])
                        n823 = Number To Decimal String(number=w1009) -> (decimal integer string=w1017:string)  [unwired: 1 in]
                        n824 = Build Array(w1010) -> (w1022:string[])
                        n825 = Build Array(w1017) -> (w1016:string[])
                        n826 = Number To Decimal String(number="平滑点数") -> (decimal integer string=w1000:string)  [unwired: 1 in]
                        n827 = Select(t="TRUE", s=w1006, f="FALSE") -> (s? t:f=w1003:string)
                        n828 = Build Array(w1000) -> (w999:string[])
                        n829 = Build Array(w1003) -> (w1002:string[])
                        n830 = Build Array(w1027, w1026, w1025, w1024, w1023, w1013, string[] ["占位符"], w1022, w1011, w1016, w1012, w1007, w1002, w999, w996) -> (w1021:string[][])
                        n831 = Transpose 2D Array(2D array=w1021) -> (transposed array=w1020:string[][])
                        n832 = Array To Spreadsheet String(delimiter (Tab)="#" ("分隔符(Tab)"), array=w1020, 3:"%s" ("格式字符串")) -> (spreadsheet string=w1008:string)
                        n833 = local write "Project Information"(w1008) -> ()
                      }
                      frame #2 {
                        n834 = local read "VNA Cal File Path:"() -> (w1057:string)
                        n835 = property on="Diff Test Items" class="LstBox (严格)"() -> ("Item Symbols"=w1054:i32[])  [unwired: 2 in, 2 out]
                        n836 = property on="Single Test Items" class="LstBox (严格)"() -> ("Item Symbols"=w1053:i32[])  [unwired: 2 in, 2 out]
                        n837 = property on="TDR Test Items" class="LstBox (严格)"() -> ("Item Symbols"=w1052:i32[])  [unwired: 2 in, 2 out]
                        n838 = property on="S-para Pair Name" class="LstBox (严格)"() -> ("Item Symbols"=w1051:i32[])  [unwired: 2 in, 2 out]
                        n839 = property on="NEXT Pair Name" class="LstBox (严格)"() -> ("Item Symbols"=w1050:i32[])  [unwired: 2 in, 2 out]
                        n840 = property on="FEXT Pair Name" class="LstBox (严格)"() -> ("Item Symbols"=w1046:i32[])  [unwired: 2 in, 2 out]
                        n841 = local read "Luxshare_P/N:"() -> (w1044:string)
                        n842 = local read "Length(mm):"() -> (w1058:string)
                        n843 = String Length(string=w1044) -> (length=w1045:i32)
                        n844 = Empty String/Path?(string/path=w1057) -> (empty?=w1055:bool)
                        n845 = Empty String/Path?(string/path=w1058) -> (empty?=w1056:bool)
                        n846 = Build Array(w1054, w1053, w1052, w1051, w1050, w1046) -> (w1049:i32[][])
                        n847 = Not(x=w1056) -> (.not. x?=w1048:bool)
                        n848 = Not(x=w1055) -> (.not. x?=w1047:bool)
                        n849 = Greater Than 0?(x=w1045) -> (x > 0?=w1043:bool)
                        n850 = call "_wmg_whetherItemsEmpty.vi"("Input"=w1049) -> ("bool"=w1059:bool)
                        n851 = local read "Spec Associate"() -> (w1038:string[][])
                        n852 = Compound Arithmetic op=AND(w1043, w1048, w1047, w1059) -> (w1042:bool)
                        n853 = local write "save?"(w1042) -> ()
                        n854 = Array To Spreadsheet String(delimiter (Tab)="#" ("分隔符(Tab)"), array=w1038, 3:"%s" ("格式字符串")) -> (spreadsheet string=w1041:string)
                        n855 = local write "Spec String"(w1041) -> ()
                      }
                      frame #3 {
                        n856 = local read "Local"() -> (w1060:bool)
                        n857 = case shown="真" w1060 {
                          frame False {
                            # "17"
                            # "16"
                            # "15"
                            # "14"
                            # "13"
                            # "11"
                            # "10"
                            # "9"
                            # "8"
                            # "7"
                            # "6"
                            # "5"
                            # "4"
                            # "3"
                            # "2"
                            # "1"
                            n858 = Format Date/Time String(time format string (%c)="%Y-%m-%d : %H:%M" ("时间格式字符串(%c)")) -> (date/time string=w1061:string)  [unwired: 2 in]
                            n859 = local read "Label Print?"() -> (w1072:bool)
                            n860 = local read "fre-save"() -> (w1079:string[])
                            n861 = local read "UserID"() -> (w1064:string)
                            n862 = Boolean To (0,1)(Boolean=w1072) -> (0, 1=w1097:i16)
                            n863 = local read "EEPROM Write/Read ?"() -> (w1073:bool)
                            n864 = local read "Sample Description:"() -> (w1093:string)
                            n865 = local read "Project Information"() -> (w1094:string)
                            n866 = Array To Spreadsheet String(delimiter (Tab)="," ("分隔符(Tab)"), array=w1079, 3:"" ("格式字符串")) -> (spreadsheet string=w1076:string)
                            n867 = local read "厂区"() -> (w1066:string)
                            n868 = Number To Decimal String(number=w1097) -> (decimal integer string=w1087:string)  [unwired: 1 in]
                            n869 = Concatenate Strings(w1064, " updated@ " ("字符串"), w1061) -> (w1063:string)
                            n870 = local read "Customer_P/N:"() -> (w1096:string)
                            n871 = local read "Switch File Path"() -> (w1071:string)
                            n872 = local read "Switch Matrix"() -> (w1089:string)
                            n873 = local read "Label Content"() -> (w1086:string)
                            n874 = local read "Length(mm):"() -> (w1091:string)
                            n875 = local read "Spec String"() -> (w1090:string)
                            n876 = call <vilib>:"Trim Whitespace.vi"("string"=w1076) -> ("trimmed string"=w1075:string)  [unwired: 1 in]
                            n877 = property on="Customer" class="Ring (严格)"() -> ("RingText.Text"=w1095:string)  [unwired: 2 in, 2 out]
                            n878 = property on="Cable AWG:" class="Ring (严格)"() -> ("RingText.Text"=w1092:string)  [unwired: 2 in, 2 out]
                            n879 = local read "FixtureNo"() -> (w1084:string)
                            n880 = local read "Label Num"() -> (w1099:string)
                            n881 = local read "Remark:"() -> (w1085:string)
                            n882 = Boolean To (0,1)(Boolean=w1073) -> (0, 1=w1098:i16)
                            n883 = local read "AutoSN"() -> (w1081:bool)
                            n884 = Number To Decimal String(number=w1098) -> (decimal integer string=w1088:string)  [unwired: 1 in]
                            n885 = Boolean To (0,1)(Boolean=w1081) -> (0, 1=w1082:i16)
                            n886 = Number To Decimal String(number=w1082) -> (decimal integer string=w1080:string)  [unwired: 1 in]
                            n887 = local read "Luxshare_P/N:"() -> (w1083:string)
                            n888 = local read "Spec File Path"() -> (w1070:string)
                            n889 = local read "Spec Points"() -> (w1069:dbl)
                            n890 = property on="System_Mode" class="Ring (严格)"() -> ("RingText.Text"=w1067:string)  [unwired: 2 in, 2 out]
                            n891 = Number To Decimal String(number=w1069) -> (decimal integer string=w1068:string)  [unwired: 1 in]
                            n892 = Build Array(w1083, w1096, w1095, w1094, w1093, w1092, w1091, w1090, w1089, w1088, w1084, w1087, w1099, w1086, w1085, w1080, w1075, w1071, w1070, w1068, w1067, w1066, w1063) -> (w1074:string[])
                            n893 = local write "Project File"(w1074) -> ()
                          }
                          frame True {
                            # "20"
                            # "19"
                            # "11"
                            # "10"
                            # "9"
                            # "8"
                            # "7"
                            # "6"
                            # "5"
                            # "4"
                            # "3"
                            # "2"
                            # "1"
                            n894 = local read "Label Print?"() -> (w1106:bool)
                            n895 = local read "fre-save"() -> (w1113:string[])
                            n896 = Boolean To (0,1)(Boolean=w1106) -> (0, 1=w1131:i16)
                            n897 = local read "EEPROM Write/Read ?"() -> (w1108:bool)
                            n898 = local read "Sample Description:"() -> (w1127:string)
                            n899 = local read "Project Information"() -> (w1128:string)
                            n900 = Array To Spreadsheet String(delimiter (Tab)="," ("分隔符(Tab)"), array=w1113, 3:"" ("格式字符串")) -> (spreadsheet string=w1110:string)
                            n901 = local read "SNType"() -> (w1107:string)
                            n902 = Number To Decimal String(number=w1131) -> (decimal integer string=w1121:string)  [unwired: 1 in]
                            n903 = local read "Customer_P/N:"() -> (w1130:string)
                            n904 = local read "Switch Matrix"() -> (w1123:string)
                            n905 = local read "Label Content"() -> (w1120:string)
                            n906 = local read "Length(mm):"() -> (w1125:string)
                            n907 = local read "Spec String"() -> (w1124:string)
                            n908 = property on="CmdType" class="Ring (严格)"() -> ("RingText.Text"=w1105:string)  [unwired: 2 in, 2 out]
                            n909 = call <vilib>:"Trim Whitespace.vi"("string"=w1110) -> ("trimmed string"=w1102:string)  [unwired: 1 in]
                            n910 = property on="Customer" class="Ring (严格)"() -> ("RingText.Text"=w1129:string)  [unwired: 2 in, 2 out]
                            n911 = property on="Cable AWG:" class="Ring (严格)"() -> ("RingText.Text"=w1126:string)  [unwired: 2 in, 2 out]
                            n912 = local read "FixtureNo"() -> (w1118:string)
                            n913 = local read "Label Num"() -> (w1133:string)
                            n914 = local read "Remark:"() -> (w1119:string)
                            n915 = local read "Switch File Path"() -> (w1103:string)
                            n916 = Boolean To (0,1)(Boolean=w1108) -> (0, 1=w1132:i16)
                            n917 = local read "AutoSN"() -> (w1115:bool)
                            n918 = Number To Decimal String(number=w1132) -> (decimal integer string=w1122:string)  [unwired: 1 in]
                            n919 = Boolean To (0,1)(Boolean=w1115) -> (0, 1=w1116:i16)
                            n920 = Number To Decimal String(number=w1116) -> (decimal integer string=w1114:string)  [unwired: 1 in]
                            n921 = local read "Luxshare_P/N:"() -> (w1117:string)
                            n922 = local read "Spec File Path"() -> (w1104:string)
                            n923 = local read "Spec Points"() -> (w1101:dbl)
                            n924 = Number To Decimal String(number=w1101) -> (decimal integer string=w1100:string)  [unwired: 1 in]
                            n925 = Build Array(w1117, w1130, w1129, w1128, w1127, w1126, w1125, w1124, w1123, w1122, w1105, w1107, w1118, w1121, w1133, w1120, w1119, w1114, w1102, w1103, w1104, w1100) -> (w1109:string[])
                            n926 = local write "Project File"(w1109) -> ()
                          }
                        }
                      }
                      frame #4 {
                        n927 = local read "save?"() -> (w1135:bool)
                        n928 = case shown="真" w1135 {
                          tunnel: w1134 -> [_ w1137]
                          frame False {
                            n929 = One Button Dialog(message="保存信息不完整" ("消息")) -> ()  [unwired: 1 in, 1 out]
